vi "Read layout.vi"(8 "error in (no error)":errorcluster, 11 "ConsoleAppender in":refnum<class "ConsoleAppender.lvclass">) -> (0 "error out":errorcluster, 2 "Lumberjack.lvlib:Layout.lvclass":refnum<class "Layout.lvclass">, 3 "ConsoleAppender out":refnum<class "ConsoleAppender.lvclass">)   [LabVIEW 2026, in "Lumberjack.lvlib" / "ConsoleAppender.lvclass"]
uses:
  ConsoleAppender.lvclass
  Layouts/Layout.lvclass/Layout.lvclass
  ConsoleAppender.lvclass/ConsoleAppender.ctl
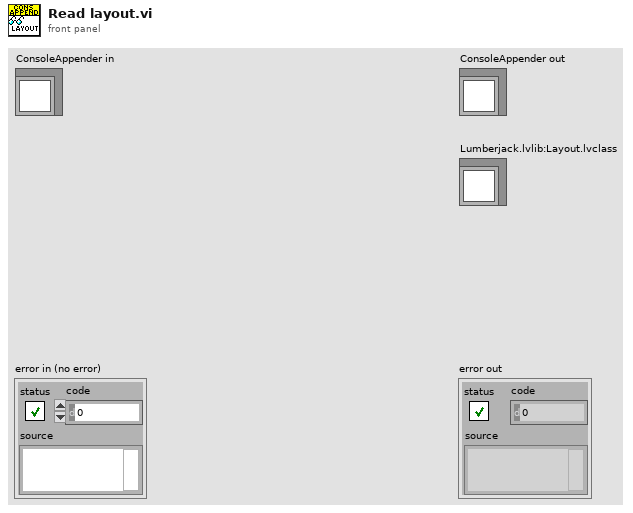
[diagram p1: front panel]
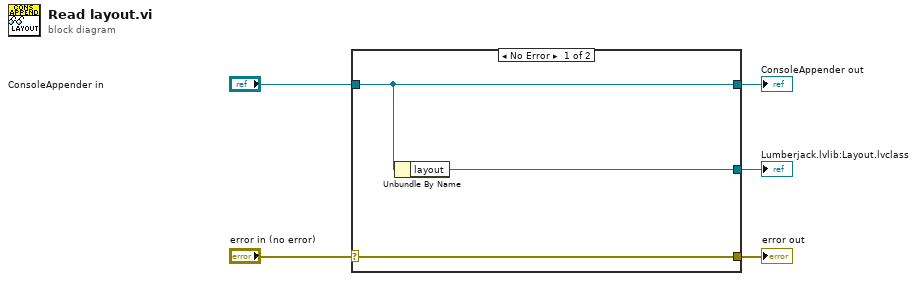
[diagram p0: block diagram]
diagram:
  n1 = case shown="No Error" "error in (no error)" {
    selector: "error in (no error)" -> [w8 w9]
    tunnel: [w8 w9] -> w4
    tunnel: [w7 w10] -> w2
    tunnel: "ConsoleAppender in" -> [w7 w10]
    tunnel: [w6 _] -> w1
    frame No Error {
      n2 = Unbundle By Name(w7) -> ("layout"=w6:refnum<class "Layout.lvclass">)
    }
    frame Error {
    }
  }
  "error out" <- w4
  "ConsoleAppender out" <- w2
  "Lumberjack.lvlib:Layout.lvclass" <- w1
